vi "One Time Surge Drop Trigger.vi"(0 "VISA Resource Name":refnum<visa-resource-name>, 11 "error in (no error)":errorcluster) -> (4 "VISA resource name out":refnum<visa-resource-name>, 15 "error out":errorcluster)   [LabVIEW 2020, in "eec 6700.lvlib"]
doc: "Triggers a one shot surge/drop in order to simulate loading or brown out conditions."
uses:
  <instrlib>/eec 6700/eec 6700.lvlib
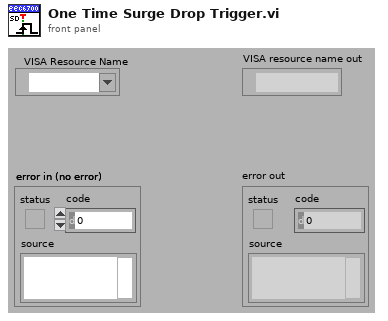
[diagram p1: front panel]
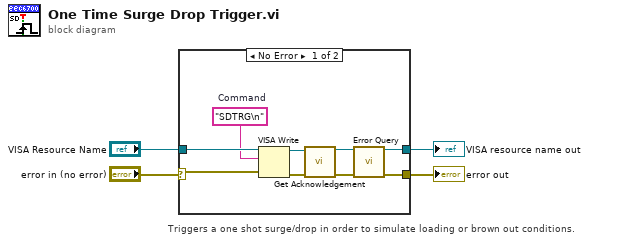
[diagram p0: block diagram]
diagram:
  # "Triggers a one shot surge/drop in order to simulate loading or brown out conditions."
  n1 = case shown="No Error" "error in (no error)" {
    selector: "error in (no error)" -> [w12 w15]
    tunnel: "VISA Resource Name" -> [w13 w14]
    tunnel: [w11 w14] -> w3
    tunnel: [w10 w15] -> w2
    frame No Error {
      w9 = "SDTRG\n"  # Command
      n2 = VISA Write(VISA resource name=w13, write buffer=w9, error in (no error)=w12) -> (VISA resource name out=w7:refnum<visa-resource-name>, error out=w6:errorcluster)  [unwired: 1 out]
      n3 = call <instrlib>:"Get Acknowledgement.vi"("VISA resource name"=w7, "error in (no error)"=w6) -> ("VISA resource name out"=w8:refnum<visa-resource-name>, "error out"=w5:errorcluster)  [unwired: 12 in]
      n4 = call <instrlib>:"Error Query.vi"("VISA resource name"=w8, "error in (no error)"=w5) -> ("VISA resource name out"=w11:refnum<visa-resource-name>, "error out"=w10:errorcluster)  [unwired: 10 in, 2 out]
    }
    frame Error {
    }
  }
  "error out" <- w2
  "VISA resource name out" <- w3
